vi "Write Numeric.vi"(8 "error in (no error)":errorcluster, 10 "Numeric":dbl, 11 "Example in":refnum<class "Example.lvclass">) -> (0 "error out":errorcluster, 3 "Example out":refnum<class "Example.lvclass">)   [LabVIEW 2015, in "Example.lvclass"]
uses:
  Example.lvclass
  Example.lvclass/Example.ctl
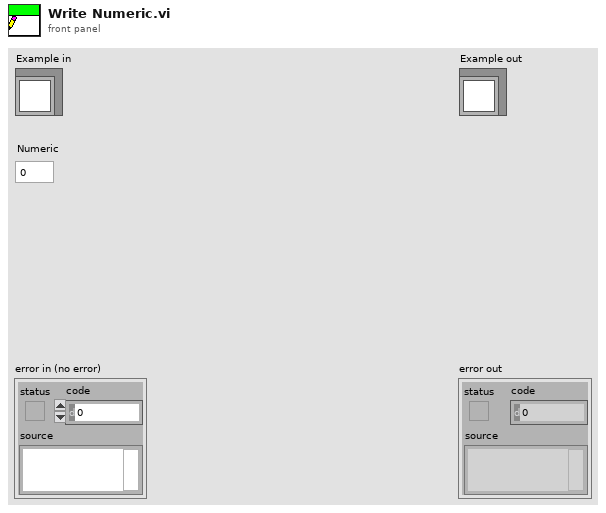
[diagram p1: front panel]
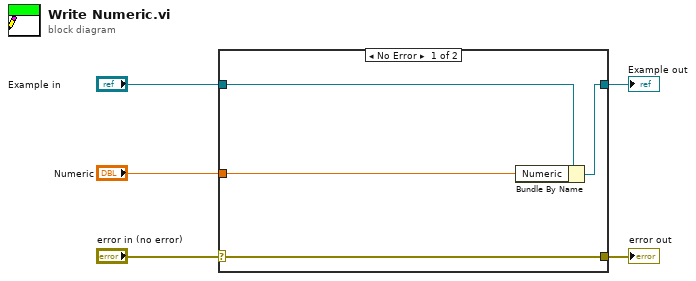
[diagram p0: block diagram]
diagram:
  n1 = case shown="No Error" "error in (no error)" {
    selector: "error in (no error)" -> [w9 w10]
    tunnel: [w9 w10] -> w4
    tunnel: [w7 w11] -> w2
    tunnel: "Example in" -> [w8 w11]
    tunnel: "Numeric" -> [w6 _]
    frame No Error {
      n2 = Bundle By Name(cluster=w8, "Numeric"=w6) -> (w7:refnum<class "Example.lvclass">)
    }
    frame Error {
    }
  }
  "error out" <- w4
  "Example out" <- w2
